vi "Convert Location to Address String.vi"(11 "Response Data":T1) -> (3 "String":string)   [LabVIEW 2020, in "NI-DCPower Source DC Voltage.lvlib"]
uses:
  NI-DCPower Source DC Voltage.lvlib
  <vilib>/MeasurementLink/MeasurementLink Discovery Client/RPC Messages/ni_measurementlink_discovery_v1_ServiceLocation.ctl
  <vilib>/MeasurementLink/MeasurementLink Discovery Client/MeasurementLink Discovery Client.lvlib
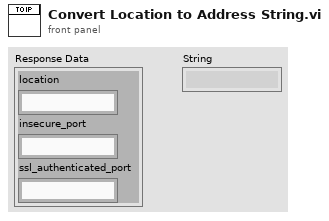
[diagram p1: front panel]
types:
  T1 = typedef "MeasurementLink Discovery Client.lvlib/ni_measurementlink_discovery_v1_ServiceLocation.ctl" = cluster{"location":string, "insecure_port":string, "ssl_authenticated_port":string}
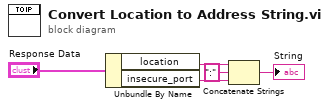
[diagram p0: block diagram]
diagram:
  n1 = Unbundle By Name("Response Data") -> ("location"=w2:string, "insecure_port"=w3:string)
  n2 = Concatenate Strings(w2, ":" ("string"), w3) -> (→"String":string)
